vi "Initialize From JSON 1.0.vi"(8 "error in (no error)":errorcluster, 11 "json":string) -> (0 "error out":errorcluster, 3 "channel configuration 1.0":T1(array[cluster]) {"string offset" format="%d bytes"})   [LabVIEW 2017, in "DSF Core.lvlib" / "Core Channels Configuration.lvclass"]
uses:
  Core Channels Configuration.lvclass
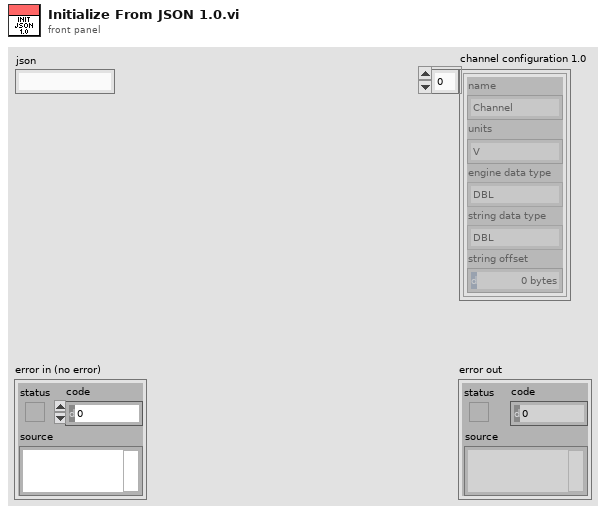
[diagram p1: front panel]
types:
  T1 = cluster{"name":string, "units":string, "engine data type":enum8{"Bool", "SGL", "DBL", "I8", "I16", "I32", "I64", "U8", "U16", "U32", "U64"}, "string data type":enum8{"Bool", "SGL", "DBL", "I8", "I16", "I32", "I64", "U8", "U16", "U32", "U64"}, "string offset":u64}[]
  T2 = cluster{"name":string, "units":string, "engine data type":u8, "string data type":u8, "string offset":u64}[]
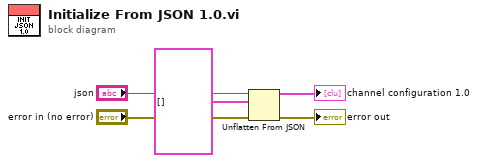
[diagram p0: block diagram]
diagram:
  n1 = Unflatten From JSON(JSON string="json", type and defaults=T2 [] ("channel configuration 1.0"), error in (no error)="error in (no error)") -> (value=→"channel configuration 1.0":T2, error out=→"error out":errorcluster)  [unwired: 4 in]
